vi "Load BaseNodeType from System Storage File.vi"(8 "error in (no error)":errorcluster, 11 "path":path) -> (0 "error out":errorcluster, 3 "BaseNodeType":refnum<k24>)   [LabVIEW 2017, in "Import Export.lvlib"]
uses:
  Import Export.lvlib
  NationalInstruments.VeriStand.SystemStorage
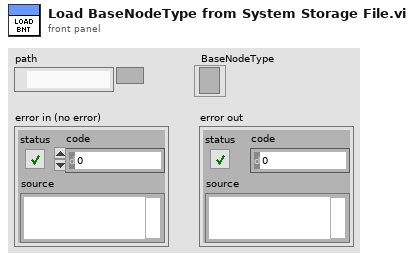
[diagram p1: front panel]
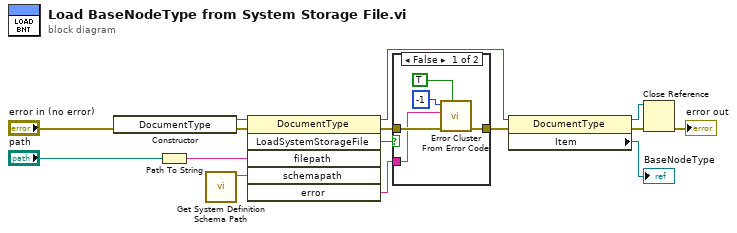
[diagram p0: block diagram]
diagram:
  n1 = constructor class="DocumentType"(error in="error in (no error)") -> (reference out=w7:refnum<k24>, error out=w6:errorcluster)  [unwired: 2 in, 1 out]
  n2 = Path To String(path="path") -> (string=w8:string)
  n3 = call "Get System Definition Schema Path.vi"() -> ("system definition schema path"=w9:string)  [unwired: 11 in]
  n4 = invoke class="DocumentType" method="LoadSystemStorageFile"(reference=w7, error in=w6, "filepath"=w8, "schemapath"=w9) -> (reference out=w14:refnum<k24>, error out=w10:errorcluster, "LoadSystemStorageFile"=w13:bool, "error"=w12:string)  [unwired: 2 in, 2 out]
  n5 = case shown="False" w13 {
    tunnel: [w18 w21] -> w11
    tunnel: w10 -> [w19 w21]
    tunnel: w12 -> [w16 _]
    frame False {
      n6 = call <vilib>:"Error Cluster From Error Code.vi"("show call chain? (False)"=TRUE, "error in (no error)"=w19, "error message (\"\")"=w16, "error code (0)"=-1) -> ("error out"=w18:errorcluster)  [unwired: 5 in]
    }
    frame True {
    }
  }
  n7 = property class="DocumentType"(reference=w14, error in=w11) -> (reference out=w5:refnum<k24>, error out=w2:errorcluster, "Item"=→"BaseNodeType":refnum<k24>)
  n8 = Close Reference(reference=w5, error in (no error)=w2) -> (error out=→"error out":errorcluster)
